vi "EMBALLAGE_BDD_ScanZebraPrinters.vi"(8 "error in (no error)":errorcluster caption="entrée d'erreur (pas d'erreur)") -> (0 "error out":errorcluster caption="sortie d'erreur", 1 "Liste Nom":string[](array[string]), 2 "Liste IP":string[](array[string]), 3 "Tableau":string[][](array[string]))   [LabVIEW 2020]
uses:
  <vilib>/Utility/file.llb/Read Delimited Spreadsheet (string).vi
  <vilib>/httpClient/LabVIEWHTTPClient.lvlib
panel:
  in  "Tab Control":enum32{"Actuel", "old"}(tab)
  out "body":string
  out "standard output":string caption="sortie standard"
  out "standard error":string caption="erreur standard"
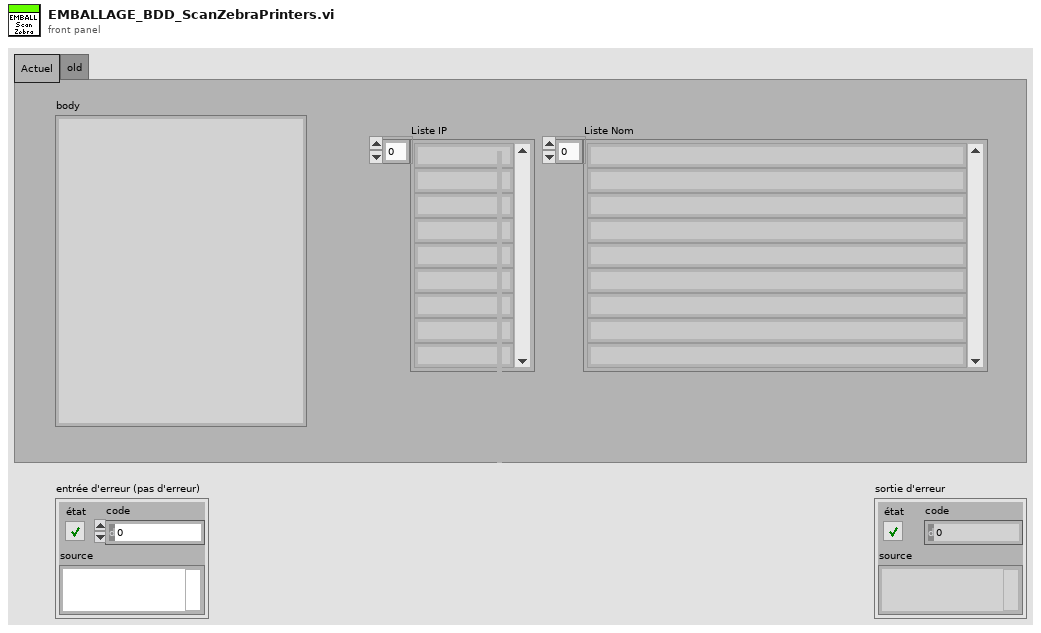
[diagram p1: front panel]
types:
  T1 = cluster{"PRINTER_NAME":string, "COMMENT":string, "IP_ADDRESS":string, "CODIF_GPAO":string}[]
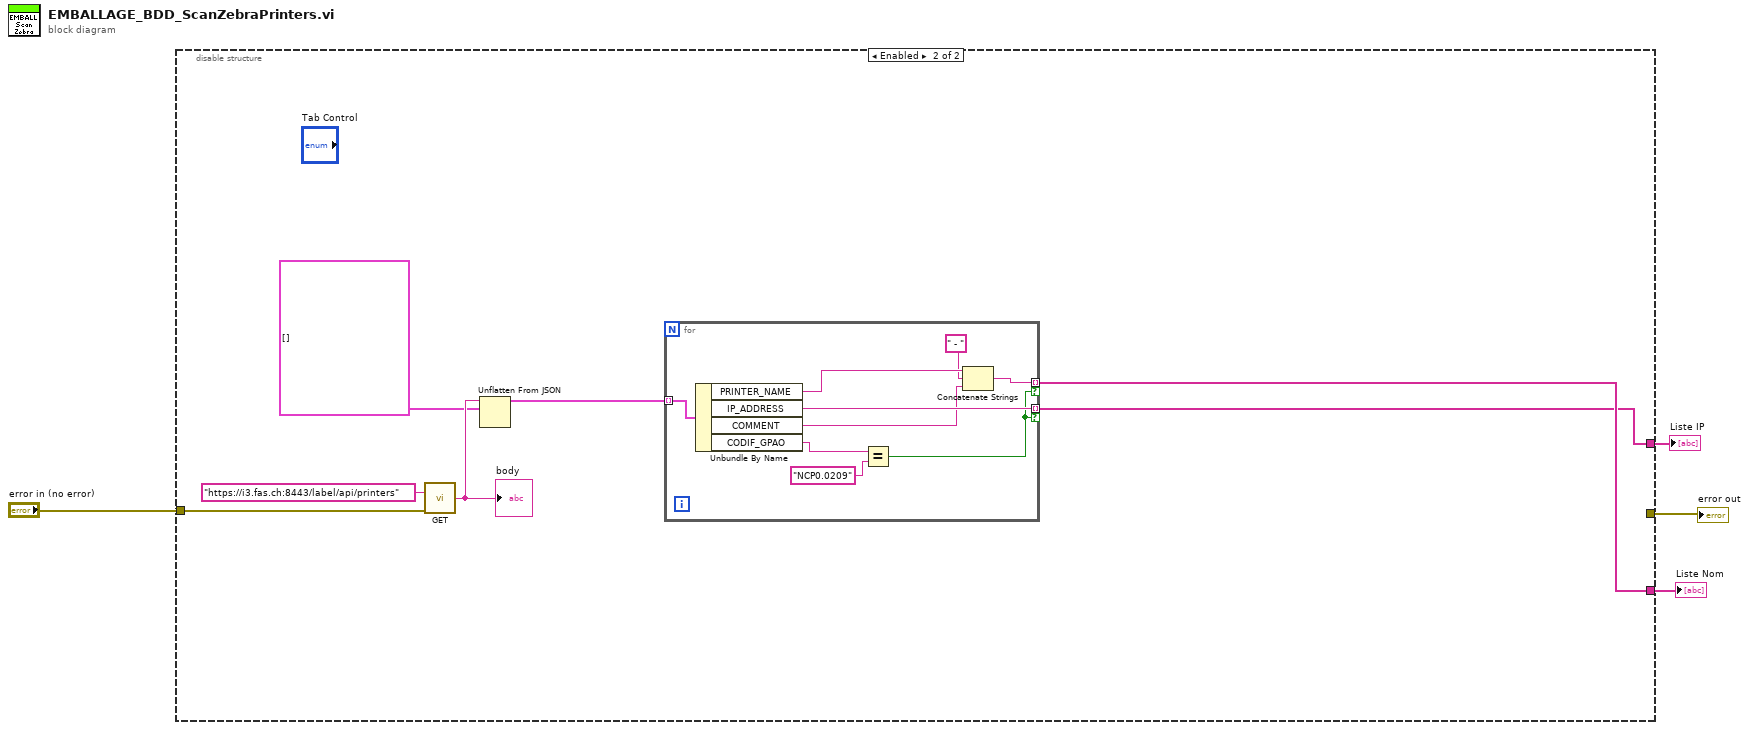
[diagram p0: block diagram]
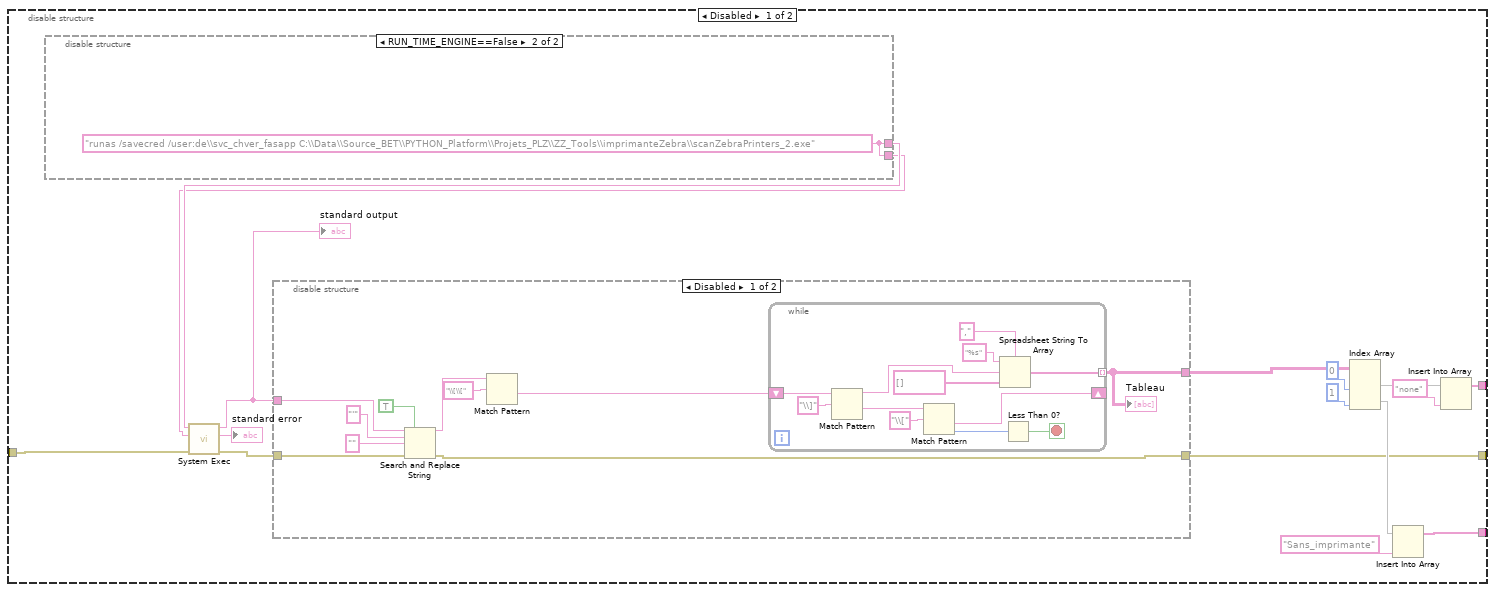
[diagram p2: hidden frame]
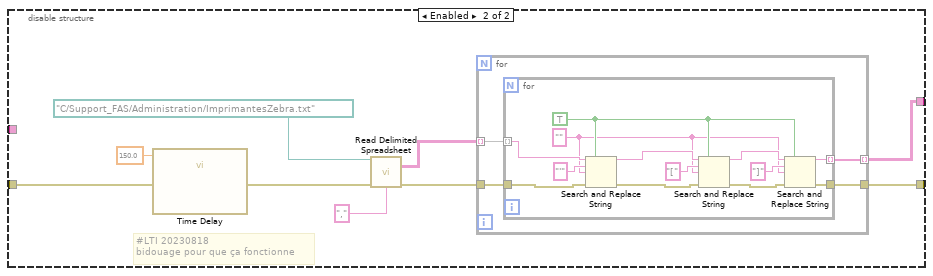
[diagram p3: hidden frame]
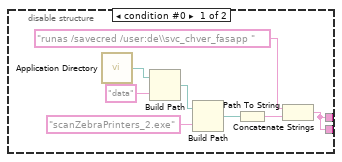
[diagram p4: hidden frame]
diagram:
  n1 = disable-structure shown="Enabled" {
    disable-tunnel: "error in (no error)" -> [w20 w83]
    disable-tunnel: [w13 w78] -> w3
    disable-tunnel: [w11 w79] -> w2
    disable-tunnel: [w5 _] -> w1
    frame Disabled {
      n2 = disable-structure shown="RUN_TIME_ENGINE==False" {
        disable-tunnel: [w69 w77] -> w15
        disable-tunnel: [w69 w77] -> w8
        frame condition #0 {
          n3 = call <vilib>:"Application Directory.vi"() -> ("Application Directory"=w72:path)
          n4 = Build Path(base path=w72, name or relative path="data" ("nom ou chemin relatif")) -> (appended path=w74:path)
          n5 = Build Path(base path=w74, name or relative path="scanZebraPrinters_2.exe" ("nom ou chemin relatif")) -> (appended path=w76:path)
          n6 = Path To String(path=w76) -> (string=w71:string)
          n7 = Concatenate Strings("runas /savecred /user:de\\svc_chver_fasapp " ("string"), w71) -> (w69:string)
        }
        frame condition #1 (active) {
          w77 = "runas /savecred /user:de\\svc_chver_fasapp C:\\Data\\Source_BET\\PYTHON_Platform\\Projets_PLZ\\ZZ_Tools\\imprimanteZebra\\scanZebraPrinters_2.exe" ("command line")
        }
      }
      n8 = call <vilib>:"System Exec.vi"("error in (no error)"=w20, "standard input"=w8, "command line"=w15) -> ("error out"=w6:errorcluster, "standard error"=→"standard error":string, "standard output"=w7:string)  [unwired: 5 in, 1 out]
      "standard output" <- w7
      n9 = disable-structure shown="Disabled" {
        disable-tunnel: [w28 w48] -> w18
        disable-tunnel: w7 -> [w27 _]
        disable-tunnel: w6 -> [w26 w49]
        disable-tunnel: [w24 w47] -> w5
        frame Disabled {
          n10 = Search and Replace String(replace all?=TRUE ("tout remplacer ? (F)"), input string=w27, search string="'" ("chaîne recherchée"), replace string="" ("chaîne de remplacement (\"\")"), error in=w26) -> (result string=w25:string, error out=w24:errorcluster)  [unwired: 3 in, 2 out]
          n11 = Match Pattern(string=w25, regular expression="\\[\\[" ("expression régulière")) -> (after substring=w29:string)  [unwired: 1 in, 3 out]
          n12 = while {
            tunnel: [w36] -> w28 mode=indexing
            shift-right: [w33] -> _
            shift-left: w29 -> [w42]
            stop <- w32 stop-if-true
            n13 = Match Pattern(string=w42, regular expression="\\]" ("expression régulière")) -> (before substring=w38:string, after substring=w35:string)  [unwired: 1 in, 2 out]
            n14 = Match Pattern(string=w35, regular expression="\\[" ("expression régulière")) -> (after substring=w33:string, offset past match=w31:i32)  [unwired: 1 in, 2 out]
            n15 = Spreadsheet String To Array(delimiter (Tab)="," ("séparateur (Tabulation)"), format string="%s" ("chaîne de format"), spreadsheet string=w38, array type (2D Dbl)=string[] []) -> (array=w36:string[])
            n16 = Less Than 0?(x=w31) -> (x < 0?=w32:bool)
          }
          "Tableau" <- w28
        }
        frame Enabled {
          # "#LTI 20230818\nbidouage pour que ça fonctionne"
          n17 = call "Time Delay"("error in (no error)"=w49, "Delay Time (s)"=150.0) -> ("error out"=w44:errorcluster)  [unwired: 9 in]
          n18 = call-poly <vilib>:"Read Delimited Spreadsheet.vi"("file path (dialog if empty)"=path "C:/Support_FAS/Administration/ImprimantesZebra.txt", "error in (no error)"=w44, "delimiter (\\t)"="," ("delimiter (\\t)")) -> ("all rows"=w51:string[][], "error out"=w50:errorcluster)  [unwired: 7 in, 4 out]
          n19 = for {
            tunnel: w51 -> [w55] mode=indexing
            tunnel: w50 -> [w54]
            tunnel: [w52] -> w47
            tunnel: [w53] -> w48 mode=indexing
            n20 = for {
              tunnel: w55 -> [w68] mode=indexing
              tunnel: w54 -> [w63]
              tunnel: [w57] -> w52
              tunnel: [w56] -> w53 mode=indexing
              w61 = TRUE ("replace all? (F)")
              w59 = "" ("replace string (\"\")")
              n21 = Search and Replace String(replace all?=w61, input string=w68, search string="'", replace string=w59, error in=w63) -> (result string=w66:string, error out=w64:errorcluster)  [unwired: 3 in, 2 out]
              n22 = Search and Replace String(replace all?=w61, input string=w66, search string="[", replace string=w59, error in=w64) -> (result string=w62:string, error out=w58:errorcluster)  [unwired: 3 in, 2 out]
              n23 = Search and Replace String(replace all?=w61, input string=w62, search string="]", replace string=w59, error in=w58) -> (result string=w56:string, error out=w57:errorcluster)  [unwired: 3 in, 2 out]
            }
          }
        }
      }
      n24 = Index Array(array=w18, index (col) #1=0 ("indice désactivé (col)"), index (col) #2=1 ("indice (col)")) -> (element #1=w14:string[], element #2=w12:string[])  [unwired: 2 in]
      n25 = Insert Into Array(array=w12, new element="Sans_imprimante") -> (w11:string[])  [unwired: 1 in]
      n26 = Insert Into Array(array=w14, new element="none" ("nouvel élément/sous-tableau")) -> (w13:string[])  [unwired: 1 in]
    }
    frame Enabled {
      n27 = call <vilib>:"GET.vi"("url"="https://i3.fas.ch:8443/label/api/printers", "error in (no error)"=w83) -> ("body"=w82:string)  [unwired: 10 in, 3 out]
      "body" <- w82
      n28 = Unflatten From JSON(JSON string=w82, type and defaults=T1 []) -> (value=w80:T1)  [unwired: 5 in, 1 out]
      n29 = for {
        tunnel: w80 -> [w93] mode=indexing
        tunnel: [w87] -> w79 mode=indexing if=w88
        tunnel: [w91] -> w78 mode=indexing if=w88
        n30 = Unbundle By Name(w93) -> ("PRINTER_NAME"=w92:string, "IP_ADDRESS"=w91:string, "COMMENT"=w86:string, "CODIF_GPAO"=w89:string)
        n31 = Equal?(x=w89, y="NCP0.0209") -> (x = y?=w88:bool)
        n32 = Concatenate Strings(w92, " - " ("string"), w86) -> (w87:string)
      }
    }
  }
  "Liste IP" <- w3
  "Liste Nom" <- w2
  "error out" <- w1
